vi "Play Musicvi.vi"(8 "error in (no error)":errorcluster, 11 "Sound LUMP IN":u8[](array[numeric])=array[17283 elements]) -> (0 "error out":errorcluster)   [LabVIEW 2014]
panel:
  in  "stop":bool
  out "Output String":string
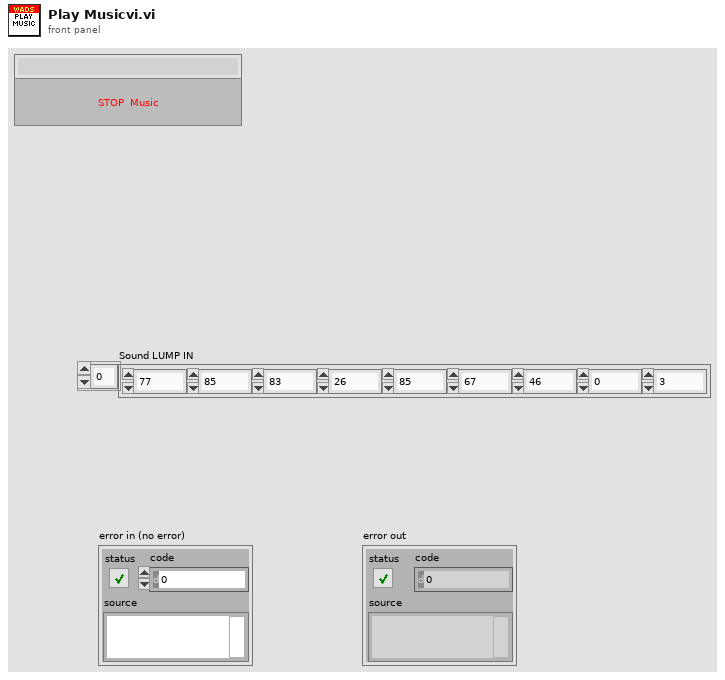
[diagram p1: front panel]
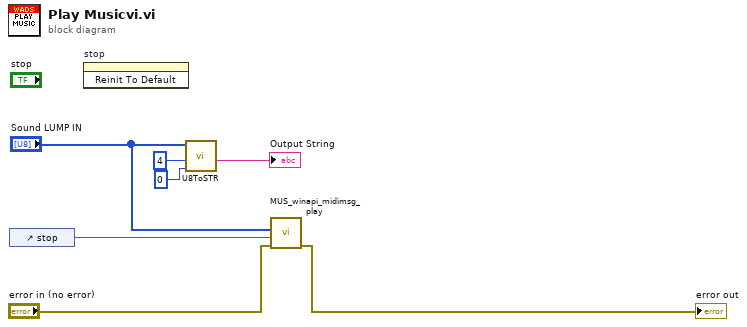
[diagram p0: block diagram]
diagram:
  n1 = control-ref of="stop"() -> (w1:refnum<vi>)
  n2 = invoke on="stop" class="Bool (strict)" method="Reinit To Default"() -> ()  [unwired: 3 in, 3 out]
  n3 = call "U8ToSTR.vi"("Index"=u32 0, "Count"=4, "Input U8 Array"="Sound LUMP IN") -> ("Output String"=→"Output String":string)  [unwired: 2 in, 2 out]
  n4 = call "MUS_winapi_midimsg_play.vi"("error in"="error in (no error)", "Stop Refnum"=w1, "MUS_data"="Sound LUMP IN") -> ("error out"=→"error out":errorcluster)  [unwired: 8 in]
